vi "Demo_BjusticeData.vi"() -> ()   [LabVIEW 2021, in "RocketPlotDemo.lvlib"]
uses:
  Demo/RocketPlotDemo.lvlib
  TypeDefs/plot load data V2.ctl
  TypeDefs/plot properties V2.ctl
  TypeDefs/plot attributes V2.ctl
  TypeDefs/Plot scale axis properties.ctl
  TypeDefs/Plot general properties.ctl
  Classes/RocketPlotHandle/SubVIs/Init Options.ctl
  TypeDefs/TimeZone.ctl
  Classes/BjusticePlotHandle/Type.ctl
  Classes/RocketPlotPanel/RocketPlotPanel.lvclass/RocketPlotPanel.ctl
  Classes/RocketPlotPanel/Read RocketPlotHandle.vi
  Classes/BjusticePlotHandle/BjusticePlotHandle.lvclass
  C:/Users/bjustice/Documents/GitHub/BluePlot/builds/RocketPlot/Source Distribution/Classes/RocketPlotHandle/RocketPlotHandle.lvclass
  Classes/RocketPlotPanel/RocketPlotPanel.lvclass
  C:/Program Files/National Instruments/LabVIEW 2021/vi.lib/IlluminatedG/IG OOPanel/OOPanel/Panel/Panel.lvclass
  Classes/RocketPlotHandle/Load PlotConfig.vi
  Classes/RocketPlotHandle/Get PlotConfig.vi
  Classes/RocketPlotHandle/RocketPlotHandle.lvclass
  RocketPlot.lvlib
  <userlib>/bjustice/Ring Buffer for Time Series Data Strict Accessor/Ring Buffer Strict Accessor.lvlib
  <vilib>/IlluminatedG/IG OOPanel/OOPanel/Manager/Manager.lvclass
panel:
  in  "load config":bool
  in  "get config":bool
  out "time to plot":dbl
  out "Subscribed names":i32(listbox)
  in  "Plot config":T1={"plots"=[], "X-axis"={"Name Label.Text"="", "Style"=0, "Tick Colors:Minor Tick Color"=0, "Tick Colors:Tick Color"=0, "Marker Colors:Text Color"=0, "Grid Colors:Major Color"=0, "Grid Colors:Minor Color"=0, "Mapping Mode"=0, "Flipped"=FALSE, "Name Label.Visible"=FALSE, "Name Label.Text Colors:Text Color"=0, "Scale Fit"=0, "Range:Maximum"=0.0, "Range:Minimum"=0.0, "Offset and Multiplier:Multiplier"=0.0, "Offset and Multiplier:Offset"=0.0, "Name Label.Font:Size"=0, "Marker.Font:Size"=0, "Uniform Marker Spacing?"=TRUE, "Format String"=""}, "Y-axes"=[], "General"={"Title"="", "Time to Plot"=1800.0, "Title.Visible"=FALSE, "Sidebar.Visible"=FALSE, "Plot Area:Colors:BG Color"=0, "X Scale.Plot Name"="", "X Scale.Use Plot Name"=FALSE}} {"General"."Time to Plot" format="%<%M:%S>t"}
  # "Documentation and user guide:"
  # "https://github.com/justiceb/BluePlot/blob/main/README.md"
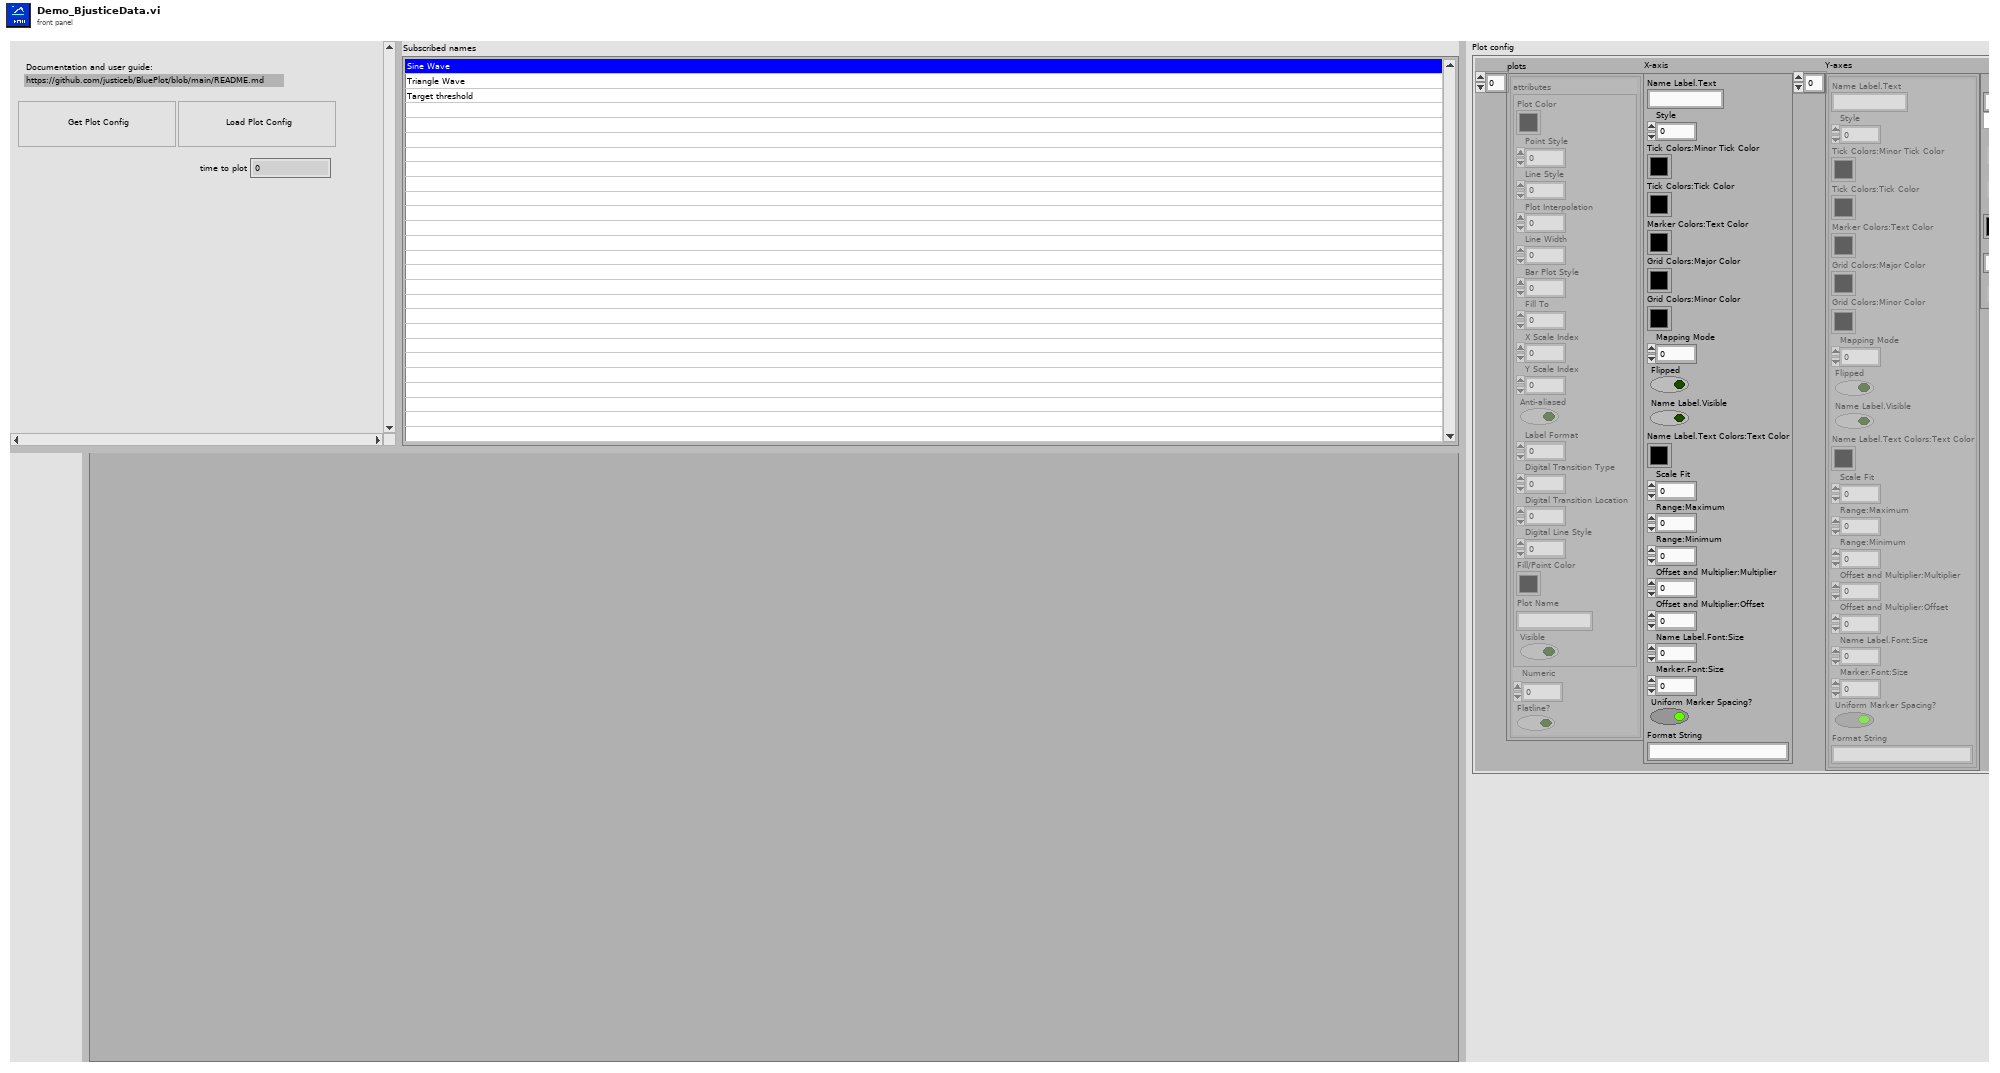
[diagram p1: front panel]
types:
  T1 = typedef "RocketPlot.lvlib/plot load data V2.ctl" = cluster{"plots":T2[], "X-axis":T4, "Y-axes":T4[], "General":T5}
  T2 = typedef "RocketPlot.lvlib/plot properties V2.ctl" = cluster{"attributes":T3, "Numeric":dbl, "Flatline?":bool}
  T3 = typedef "RocketPlot.lvlib/plot attributes V2.ctl" = cluster{"Plot Color":u32, "Point Style":u8, "Line Style":u8, "Plot Interpolation":u8, "Line Width":u8, "Bar Plot Style":u8, "Fill To":i16, "X Scale Index":u32, "Y Scale Index":u32, "Anti-aliased":bool, "Label Format":u8, "Digital Transition Type":u8, "Digital Transition Location":u8, "Digital Line Style":u8, "Fill/Point Color":u32, "Plot Name":string, "Visible":bool}
  T4 = typedef "RocketPlot.lvlib/Plot scale axis properties.ctl" = cluster{"Name Label.Text":string, "Style":u8, "Tick Colors:Minor Tick Color":u32, "Tick Colors:Tick Color":u32, "Marker Colors:Text Color":u32, "Grid Colors:Major Color":u32, "Grid Colors:Minor Color":u32, "Mapping Mode":u8, "Flipped":bool, "Name Label.Visible":bool, "Name Label.Text Colors:Text Color":u32, "Scale Fit":u8, "Range:Maximum":dbl, "Range:Minimum":dbl, "Offset and Multiplier:Multiplier":dbl, "Offset and Multiplier:Offset":dbl, "Name Label.Font:Size":u32, "Marker.Font:Size":u32, "Uniform Marker Spacing?":bool, "Format String":string}
  T5 = typedef "RocketPlot.lvlib/Plot general properties.ctl" = cluster{"Title":string, "Time to Plot":dbl, "Title.Visible":bool, "Sidebar.Visible":bool, "Plot Area:Colors:BG Color":u32, "X Scale.Plot Name":string, "X Scale.Use Plot Name":bool}
  T6 = typedef "BjusticePlotHandle.lvclass/Type.ctl" = enum16{"1PLOT", "MPLOT"}
  T7 = typedef "RocketPlotHandle.lvclass/Init Options.ctl" = cluster{"UI visible?":bool, "Update rate (ms)":u32, "Sidebar.Visible":bool, "time to plot (init)":dbl, "time to plot (max)":dbl, "config file start path":path, "Title.Visible":bool, "Title":string, "TimeZone":T8}
  T8 = typedef "RocketPlot.lvlib/TimeZone.ctl" = enum16{"UTC", "Local"}
  T9 = typedef "Ring Buffer Strict Accessor.lvlib/RingBufferHandle.ctl" = cluster{"Ring buffer DVR":refnum<data-value>, "Data Type":T10, "Size(s)":i32[], "Endianess":T11, "Buffer Size (#timestamps) [init]":i32}
  T10 = typedef "Ring Buffer Strict Accessor.lvlib/DataType.ctl" = enum16{"uint8", "uint16", "uint32", "uint64", "int8", "int16", "int32", "int64", "float", "double", "extended"}
  T11 = typedef "Ring Buffer Strict Accessor.lvlib/Endianess.ctl" = enum16{"big-endian", "little-endian"}
  T12 = cluster{"subscribed names":refnum<user-event>, "time to plot":refnum<user-event>}
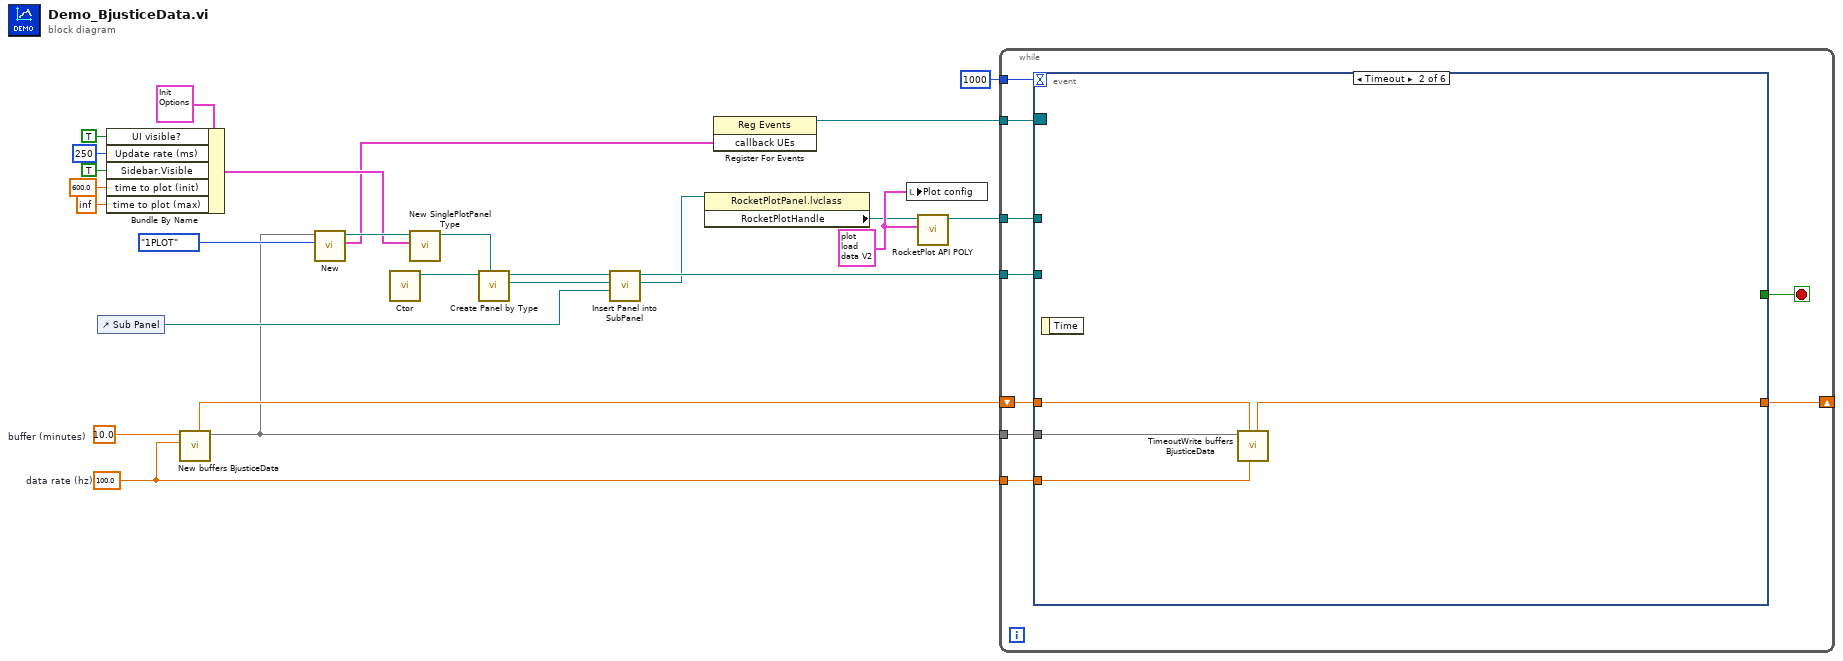
[diagram p0: block diagram]
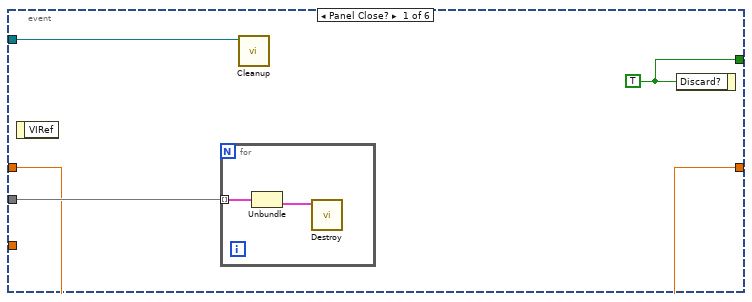
[diagram p2: hidden frame]
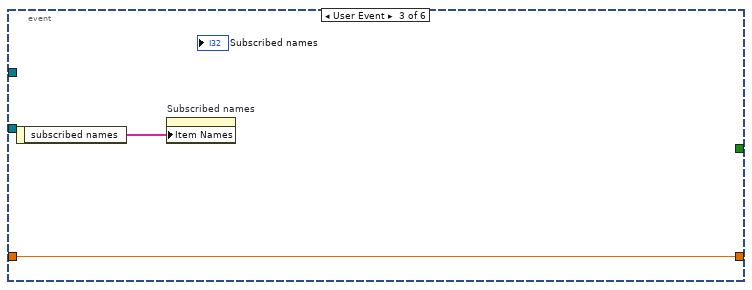
[diagram p3: hidden frame]
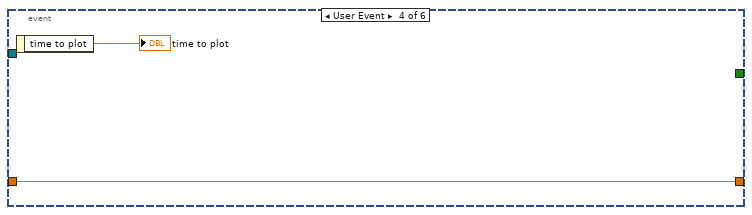
[diagram p4: hidden frame]
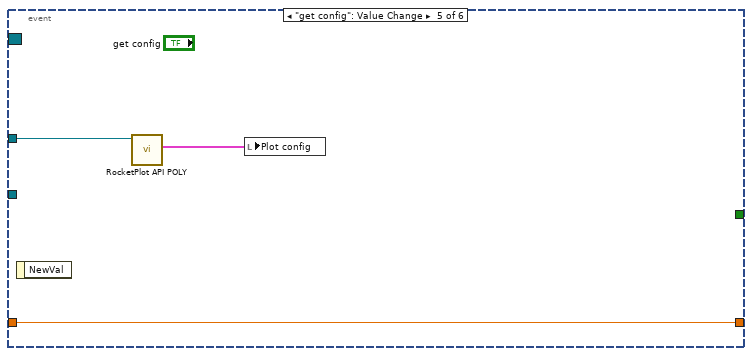
[diagram p5: hidden frame]
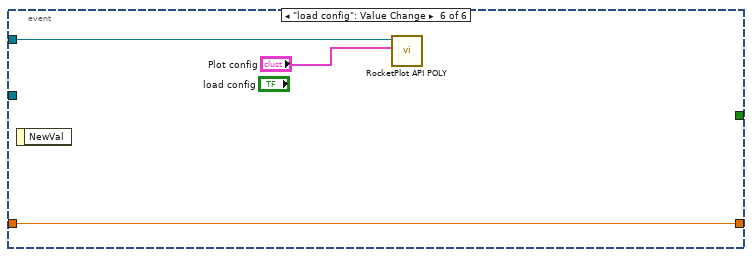
[diagram p6: hidden frame]
diagram:
  w18 = T1 {"plots"=[{"attributes"={"Plot Color"=16711680, "Point Style"=0, "Line Style"=0, "Plot Interpolation"=2, "Line Width"=0, "Bar Plot Style"=0, "Fill To"=-1, "X Scale Index"=0, "Y Scale Index"=0, "Anti-aliased"=FALSE, "Label Format"=3, "Digital Transition Type"=0, "Digital Transition Location"=2, "Digital Line Style"=1, "Fill/Point Color"=16711680, "Plot Name"="Sine Wave", "Visible"=TRUE}, "Numeric"=0.0, "Flatline?"=FALSE}, {"attributes"={"Plot Color"=4387583, "Point Style"=0, "Line Style"=0, "Plot Interpolation"=2, "Line Width"=0, "Bar Plot Style"=0, "Fill To"=-1, "X Scale Index"=0, "Y Scale Index"=1, "Anti-aliased"=FALSE, "Label Format"=3, "Digital Transition Type"=0, "Digital Transition Location"=2, "Digital Line Style"=1, "Fill/Point Color"=4387583, "Plot Name"="Triangle Wave", "Visible"=TRUE}, "Numeric"=0.0, "Flatline?"=FALSE}, {"attributes"={"Plot Color"=16722671, "Point Style"=0, "Line Style"=0, "Plot Interpolation"=2, "Line Width"=5, "Bar Plot Style"=0, "Fill To"=-1, "X Scale Index"=0, "Y Scale Index"=0, "Anti-aliased"=FALSE, "Label Format"=3, "Digital Transition Type"=0, "Digital Transition Location"=2, "Digital Line Style"=1, "Fill/Point Color"=16722671, "Plot Name"="Target threshold", "Visible"=TRUE}, "Numeric"=0.6, "Flatline?"=TRUE}, {"attributes"={"Plot Color"=16860, "Point Style"=0, "Line Style"=0, "Plot Interpolation"=2, "Line Width"=0, "Bar Plot Style"=0, "Fill To"=-1, "X Scale Index"=0, "Y Scale Index"=0, "Anti-aliased"=FALSE, "Label Format"=3, "Digital Transition Type"=0, "Digital Transition Location"=2, "Digital Line Style"=1, "Fill/Point Color"=16860, "Plot Name"="", "Visible"=TRUE}, "Numeric"=0.0, "Flatline?"=FALSE}], "X-axis"={"Name Label.Text"="Time (s)", "Style"=0, "Tick Colors:Minor Tick Color"=16777216, "Tick Colors:Tick Color"=3684408, "Marker Colors:Text Color"=16448250, "Grid Colors:Major Color"=3684408, "Grid Colors:Minor Color"=16777216, "Mapping Mode"=0, "Flipped"=FALSE, "Name Label.Visible"=TRUE, "Name Label.Text Colors:Text Color"=16448250, "Scale Fit"=2, "Range:Maximum"=3757348740.0, "Range:Minimum"=3757348080.0, "Offset and Multiplier:Multiplier"=1.0, "Offset and Multiplier:Offset"=0.0, "Name Label.Font:Size"=15, "Marker.Font:Size"=15, "Uniform Marker Spacing?"=TRUE, "Format String"="%<%H:%M:%S>T"}, "Y-axes"=[{"Name Label.Text"="Left Axis", "Style"=0, "Tick Colors:Minor Tick Color"=16777216, "Tick Colors:Tick Color"=3684408, "Marker Colors:Text Color"=16448250, "Grid Colors:Major Color"=3684408, "Grid Colors:Minor Color"=16777216, "Mapping Mode"=0, "Flipped"=FALSE, "Name Label.Visible"=FALSE, "Name Label.Text Colors:Text Color"=16448250, "Scale Fit"=2, "Range:Maximum"=1.0, "Range:Minimum"=-1.0, "Offset and Multiplier:Multiplier"=1.0, "Offset and Multiplier:Offset"=0.0, "Name Label.Font:Size"=15, "Marker.Font:Size"=15, "Uniform Marker Spacing?"=TRUE, "Format String"="%#_g"}, {"Name Label.Text"="Right Axis", "Style"=0, "Tick Colors:Minor Tick Color"=16777216, "Tick Colors:Tick Color"=3684408, "Marker Colors:Text Color"=16448250, "Grid Colors:Major Color"=3684408, "Grid Colors:Minor Color"=16777216, "Mapping Mode"=0, "Flipped"=FALSE, "Name Label.Visible"=FALSE, "Name Label.Text Colors:Text Color"=16448250, "Scale Fit"=0, "Range:Maximum"=1.0, "Range:Minimum"=-2.0, "Offset and Multiplier:Multiplier"=1.0, "Offset and Multiplier:Offset"=0.0, "Name Label.Font:Size"=15, "Marker.Font:Size"=15, "Uniform Marker Spacing?"=TRUE, "Format String"="%#_g"}], "General"={"Title"="Title", "Time to Plot"=600.0, "Title.Visible"=TRUE, "Sidebar.Visible"=TRUE, "Plot Area:Colors:BG Color"=0, "X Scale.Plot Name"="", "X Scale.Use Plot Name"=FALSE}} ("Plot config")
  w15 = 100.0  # data rate (hz)
  w17 = 10.0  # buffer (minutes)
  n1 = control-ref of="Sub Panel"() -> (w8:refnum<vi>)
  n2 = Bundle By Name(cluster=T7 {"UI visible?"=TRUE, "Update rate (ms)"=250, "Sidebar.Visible"=TRUE, "time to plot (init)"=600.0, "time to plot (max)"=inf, "config file start path"=path "", "Title.Visible"=TRUE, "Title"="Title", "TimeZone"=enum."Local"} ("Init options"), "UI visible?"=TRUE, "Update rate (ms)"=u32 250, "Sidebar.Visible"=TRUE ("visible sidebar?"), "time to plot (init)"=600.0, "time to plot (max)"=inf) -> (w11:T7)
  n3 = call "New buffers BjusticeData.vi"("data rate (hz)"=w15, "buffer (minutes)"=w17) -> ("Map"=w1:map{string, T9}, "last timestamp"=w14:dbl)  [unwired: 8 in]
  n4 = call "New.vi"("Type"=Type."1PLOT", "ChannelMap"=w1) -> ("callback UEs"=w3:T12, "StokePlotHandle out"=w12:refnum<class "BjusticePlotHandle.lvclass">)  [unwired: 7 in, 1 out]
  n5 = call <vilib>:"Ctor.vi"() -> ("Manager out"=w13:refnum<class "Manager.lvclass">)  [unwired: 10 in, 1 out]
  n6 = call "New SinglePlotPanel Type.vi"("Init options"=w11, "BluePlotHandle"=w12) -> ("SinglePlotPanel out"=w10:refnum<class "RocketPlotPanel.lvclass">)  [unwired: 8 in, 1 out]
  n7 = call <vilib>:"Create Panel by Type.vi"("Panel Type"=w10, "Manager in"=w13) -> ("Panel"=w7:refnum<class "RocketPlotPanel.lvclass">, "Manager out"=w9:refnum<class "Manager.lvclass">)  [unwired: 7 in, 1 out]
  n8 = call <vilib>:"Insert Panel into SubPanel.vi"("SubPanel"=w8, "Panel In"=w7, "Manager in"=w9) -> ("Panel"=w2:refnum<class "RocketPlotPanel.lvclass">, "Manager out"=w6:refnum<class "Manager.lvclass">)  [unwired: 6 in, 1 out]
  n9 = property class="RocketPlotPanel.lvclass"(reference=w2) -> ("RocketPlotHandle"=w5:refnum<class "RocketPlotHandle.lvclass">)  [unwired: 1 in, 2 out]
  n10 = register-events(w3) -> (reference out=w26:refnum<event-registration>)  [unwired: 2 in, 1 out]
  n11 = local write "Plot config"(w18) -> ()
  n12 = call-poly "RocketPlot API POLY.vi"("Plot config"=w18, "BluePlotHandle in"=w5) -> ("BluePlotHandle out"=w19:refnum<class "RocketPlotHandle.lvclass">)  [unwired: 8 in, 1 out]
  n13 = while {
    tunnel: w19 -> [w35]
    tunnel: w26 -> [w33]
    tunnel: w1 -> [w32]
    tunnel: 1000 ("period (ms)") -> [w31]
    shift-right: [w29] -> _
    shift-left: w14 -> [w30]
    tunnel: w15 -> [w28]
    tunnel: w6 -> [w27]
    stop <- w34 stop-if-true
    n14 = event shown="[1] Timeout" {
      selector: w33 -> [_ _ _ _ _ _]
      dyn-events: _ -> [_ _ _ _ _ _]
      timeout: w31 -> [_ _ _ _ _ _]
      tunnel: w35 -> [_ _ _ _ w52 w55]
      tunnel: [w38 _ _ _ _ _] -> w34
      tunnel: w32 -> [w39 w45 _ _ _ _]
      tunnel: w30 -> [w37 w44 w46 w48 w50 w53]
      tunnel: [w37 w43 w46 w48 w50 w53] -> w29
      tunnel: w28 -> [_ w42 _ _ _ _]
      tunnel: w27 -> [w36 _ _ _ _ _]
      event Panel Close? {
        w38 = TRUE ("Discard?")
        n15 = event-data() -> ()  [unwired: 1 in, 1 out]
        n16 = for {
          tunnel: w39 -> [w41] mode=indexing
          n17 = Unbundle(w41) -> ("Ring Buffer"=w40:T9)  [unwired: 1 out]
          n18 = call <userlib>:"Destroy.vi"("Ring Buffer"=w40) -> ()  [unwired: 10 in, 1 out]
        }
        n19 = call <vilib>:"Cleanup.vi"("Manager in"=w36) -> ()  [unwired: 8 in, 3 out]
        n20 = event-data("Discard?"=w38) -> ()  [unwired: 1 in, 1 out]
      }
      event Timeout {
        n21 = event-data() -> ()  [unwired: 1 in, 1 out]
        n22 = call "TimeoutWrite buffers BjusticeData.vi"("data rate (hz)"=w42, "previous timestamp"=w44, "Map"=w45) -> ("current timestamp"=w43:dbl)  [unwired: 8 in]
      }
      event User Event {
        n23 = event-data() -> ("subscribed names"=w47:string[])  [unwired: 1 in]
        n24 = property on="Subscribed names" class="LstBox (strict)"("Item Names"=w47) -> ()  [unwired: 2 in, 2 out]
      }
      event User Event {
        n25 = event-data() -> ("time to plot"=→"time to plot":dbl)  [unwired: 1 in]
      }
      event "get config": Value Change {
        n26 = event-data() -> ()  [unwired: 1 in, 1 out]
        n27 = call-poly "RocketPlot API POLY.vi"("BluePlotHandle in"=w52) -> ("Plot config"=w51:T1)  [unwired: 8 in, 2 out]
        n28 = local write "Plot config"(w51) -> ()
      }
      event "load config": Value Change {
        n29 = event-data() -> ()  [unwired: 1 in, 1 out]
        n30 = call-poly "RocketPlot API POLY.vi"("Plot config"="Plot config", "BluePlotHandle in"=w55) -> ()  [unwired: 8 in, 2 out]
      }
    }
  }
